vi "PicoScopeospaGetValuesOverlapped.vi"(5 "Segment Range":T1 {"toSegmentIndex" format="%.4p"; "fromSegmentIndex" format="%.4p"}, 7 "Buffer and Transfer Settings":T2={"startIndex"=0, "Samples"=1000, "Down Sample Ratio"=1, "Down-Sample Mode"=1} {"Down-Sample Mode" items=["RAW none"=2147483648, "None"=0, "Aggregate"=1, "Decimate"=2, "Average"=4]; "Down Sample Ratio" step=1; "Samples" format="%_6p"}, 8 "error in (no error)":errorcluster, 11 "handle in":i16) -> (0 "error out":errorcluster, 3 "handle out":i16, 4 "Pointer to Overflow":u64[](array[numeric]), 6 "noOfSamples":u64)   [LabVIEW 2010]
doc: "Calls GetValuesOverlapped"
uses:
  psospa.dll
  shared/Segment Range.ctl
  shared/Buffer and Transfer Settings.ctl
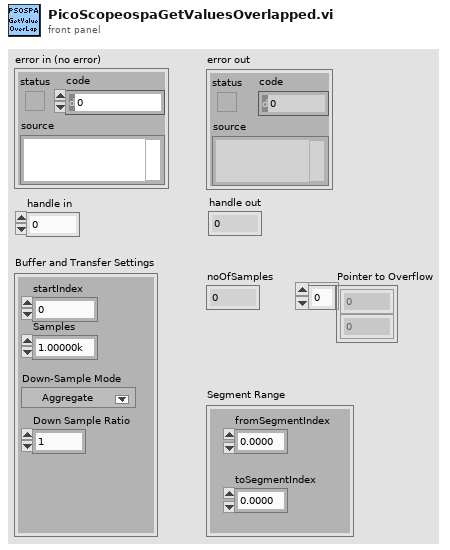
[diagram p1: front panel]
types:
  T1 = typedef "Segment Range.ctl" = cluster{"fromSegmentIndex":u64, "toSegmentIndex":u64}
  T2 = typedef "Buffer and Transfer Settings.ctl" = cluster{"startIndex":u64, "Samples":u64, "Down Sample Ratio":u64, "Down-Sample Mode":u32}
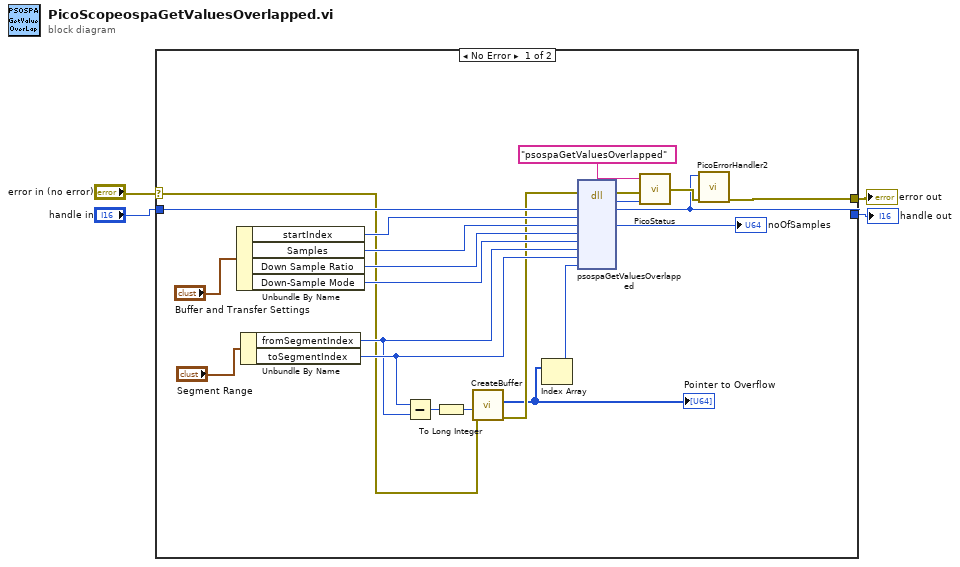
[diagram p0: block diagram]
diagram:
  n1 = case shown="No Error" "error in (no error)" {
    selector: "error in (no error)" -> [w8 w27]
    tunnel: "handle in" -> [w17 w28]
    tunnel: [w15 w28] -> w4
    tunnel: [w16 w27] -> w3
    frame No Error {
      n2 = Unbundle By Name("Buffer and Transfer Settings") -> ("startIndex"=w18:u64, "Samples"=w26:u64, "Down Sample Ratio"=w23:u64, "Down-Sample Mode"=w24:u32)
      n3 = Unbundle By Name("Segment Range") -> ("fromSegmentIndex"=w11:u64, "toSegmentIndex"=w12:u64)
      n4 = Subtract(x=w12, y=w11) -> (x-y=w10:u64)
      n5 = To Long Integer(number=w10) -> (32bit integer=w9:i32)
      n6 = call "CreateBuffer.vi"("error in (no error)"=w8, "Buffer size"=w9) -> ("error out"=w7:errorcluster, "Pointer and BufferSize"=w6:u64[])  [unwired: 8 in]
      "Pointer to Overflow" <- w6
      n7 = Index Array(array=w6) -> (element=w5:u64)  [unwired: 1 in]
      n8 = dll-call lib="psospa.dll" fn="psospaGetValuesOverlapped" ("ps3000.dll:_ps3000_open_unit@0")(error in=w7, "handle"=w17, "startIndex"=w18, "noOfSamples"=w26, "downSampleRatio"=w23, "downSampleRatioMode"=w24, "fromSegmentIndex"=w11, "toSegmentIndex"=w12, "overflow"=w5) -> (error out=w22:errorcluster, "PICO_STATUS"=w21:u32, "handle"=w15:i16, "noOfSamples"=→"noOfSamples":u64)  [unwired: 8 in, 1 out]
      n9 = call "PicoStatus.vi"("PICO STATUS"=w21, "error in"=w22, "source"="psospaGetValuesOverlapped") -> ("error out"=w25:errorcluster)
      n10 = call "PicoErrorHandler2.vi"("error in (no error)"=w25, "handle In"=w15) -> ("error out"=w16:errorcluster)  [unwired: 9 in]
    }
    frame Error {
    }
  }
  "error out" <- w3
  "handle out" <- w4
